vi "Base Error Offset.vi"() -> (3 "base error offset":i32)   [LabVIEW 2017, in "DSF Core.lvlib" / "Interface.lvclass"]
uses:
  Interface.lvclass
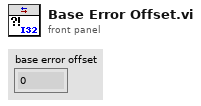
[diagram p1: front panel]
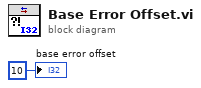
[diagram p0: block diagram]
diagram:
  "base error offset" <- 10 ("base error code")
